vi "vbMSCOMM.vi"(0 "端口号":string="COM7", 5 "Send Delay(ms)":string="100", 7 "Send Data":string="AT\r\n", 9 "Data Return":string="OK", 11 "cycle times":string="3") -> (4 "result":bool, 8 "Rec Data":string)   [LabVIEW 2013]
panel:
  out "字符串":string
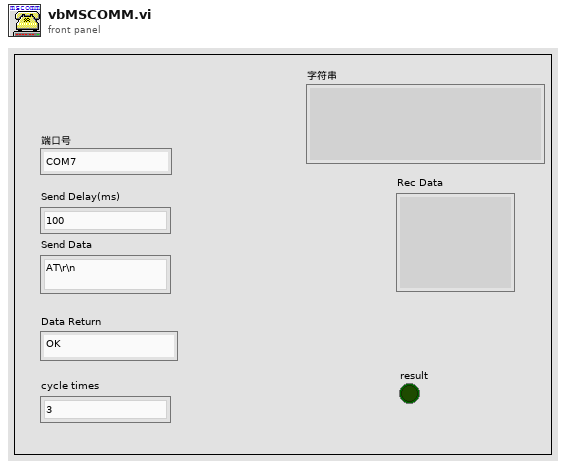
[diagram p1: front panel]
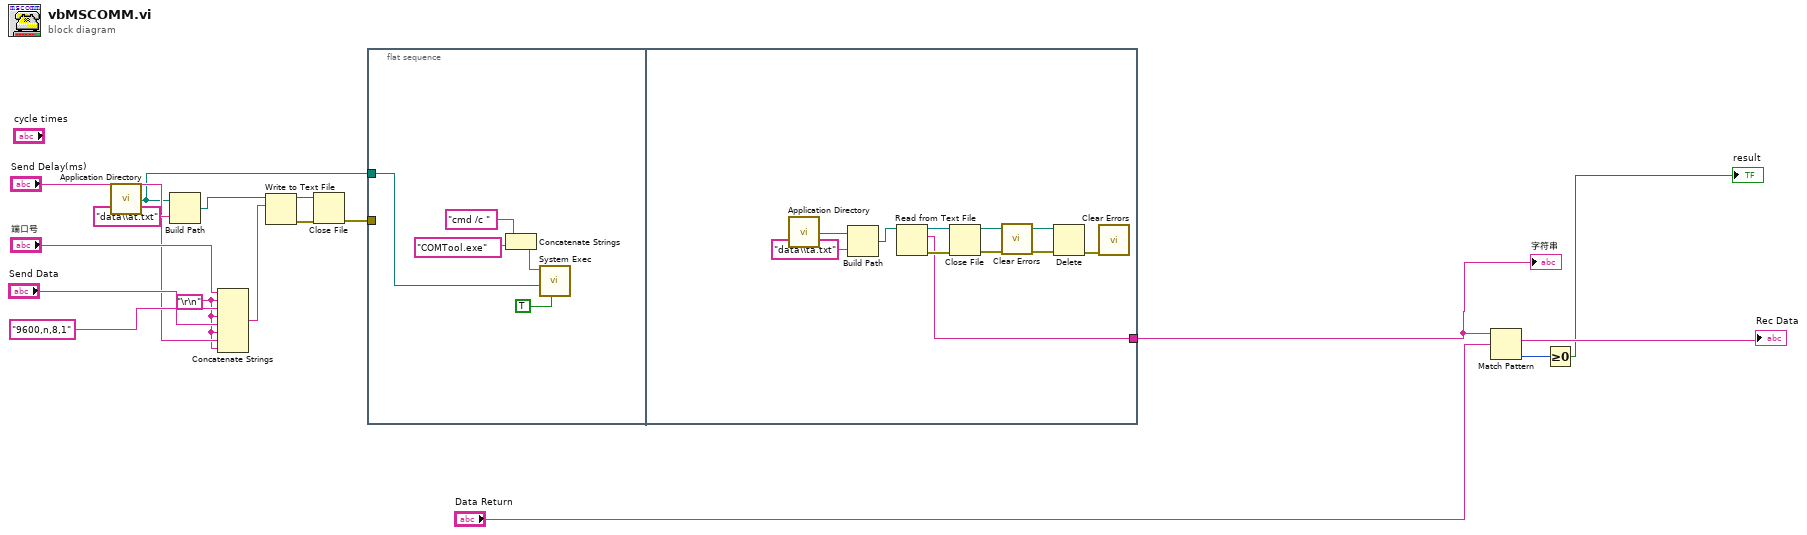
[diagram p0: block diagram]
diagram:
  w8 = "\r\n"
  n1 = call <vilib>:"Application Directory.vi"() -> ("Application Directory"=w1:path)
  n2 = Build Path(base path=w1, name or relative path="data\\at.txt" ("名称或相对路径")) -> (appended path=w2:path)
  n3 = Concatenate Strings("端口号", w8, "9600,n,8,1", w8, "Send Data", w8, "Send Delay(ms)", w8) -> (w7:string)
  n4 = Write to Text File(file (use dialog)=w2, text=w7) -> (refnum out=w4:refnum<file>, error out=w6:errorcluster)  [unwired: 2 in, 1 out]
  n5 = Close File(refnum=w4, error in=w6) -> (error out=w5:errorcluster)  [unwired: 1 out]
  n6 = flat-sequence {
    tunnel: w5 -> [_]
    tunnel: w1 -> [w18]
    tunnel: [w26] -> w3
    frame #0 {
      n7 = Concatenate Strings("cmd /c " ("command line"), "COMTool.exe") -> (w20:string)
      n8 = call <vilib>:"System Exec.vi"("run minimized? (F)"=TRUE, "working directory"=w18, "command line"=w20) -> ()  [unwired: 5 in, 4 out]
    }
    frame #1 {
      n9 = call <vilib>:"Application Directory.vi"() -> ("Application Directory"=w31:path)
      n10 = Build Path(base path=w31, name or relative path="data\\ta.txt" ("名称或相对路径")) -> (appended path=w30:path)
      n11 = Read from Text File(file (use dialog)=w30) -> (refnum out=w28:refnum<file>, text=w26:string, error out=w29:errorcluster)  [unwired: 3 in, 1 out]
      n12 = Close File(refnum=w28, error in=w29) -> (path=w24:path, error out=w27:errorcluster)
      n13 = call <vilib>:"Clear Errors.vi"("error in (no error)"=w27) -> ("error out"=w25:errorcluster)  [unwired: 6 in]
      n14 = Delete(path (use dialog)=w24, error in=w25) -> (error out=w23:errorcluster)  [unwired: 3 in, 2 out]
      n15 = call <vilib>:"Clear Errors.vi"("error in (no error)"=w23) -> ()  [unwired: 6 in, 1 out]
    }
  }
  n16 = Match Pattern(string=w3, regular expression="Data Return") -> (match substring=→"Rec Data":string, offset past match=w14:i32)  [unwired: 1 in, 2 out]
  n17 = Greater Or Equal To 0?(x=w14) -> (x >= 0?=→"result":bool)
  "字符串" <- w3
